vi "临时授权.vi"() -> (3 "授权成功":bool)   [LabVIEW 2019]
panel:
  out "不合格信息":string
  in  "授权":bool
  in  "密码":string
  in  "用户名":string(combo)
  # "产品检测不合格！\n程序已锁定！请联系管理员解除锁定！"
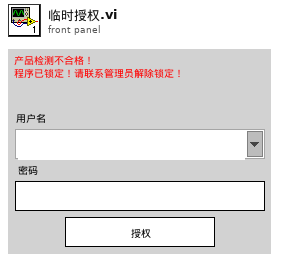
[diagram p1: front panel]
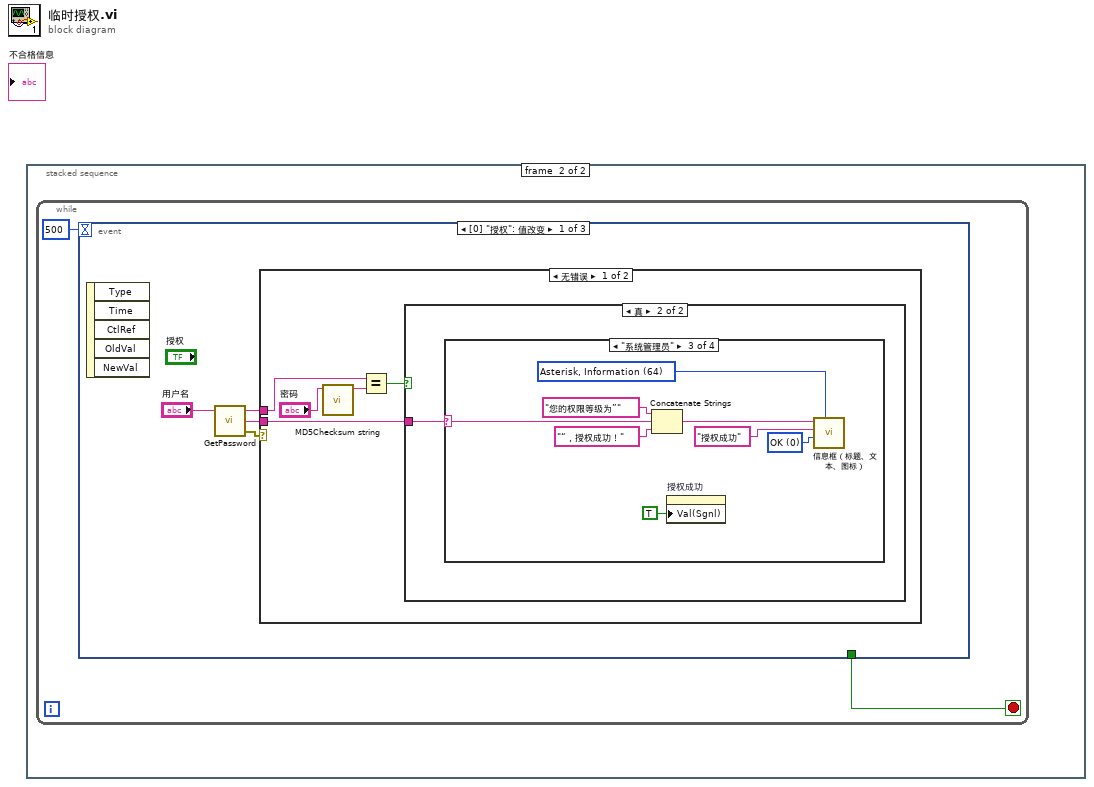
[diagram p0: block diagram]
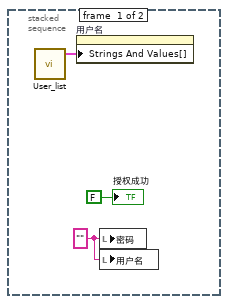
[diagram p2: hidden frame]
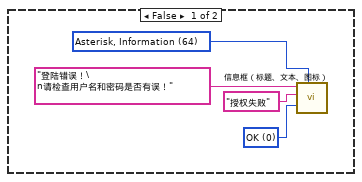
[diagram p3: hidden frame]
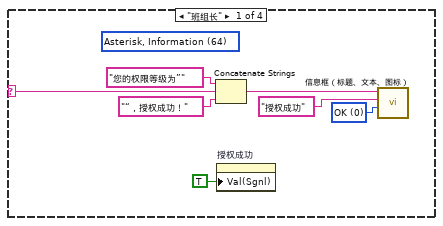
[diagram p4: hidden frame]
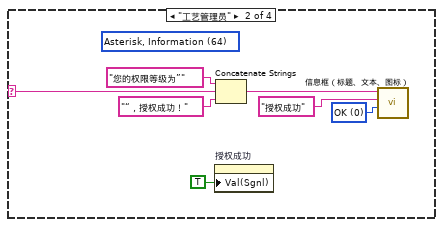
[diagram p5: hidden frame]
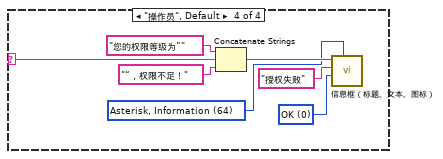
[diagram p6: hidden frame]
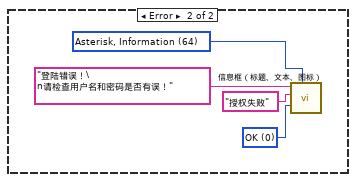
[diagram p7: hidden frame]
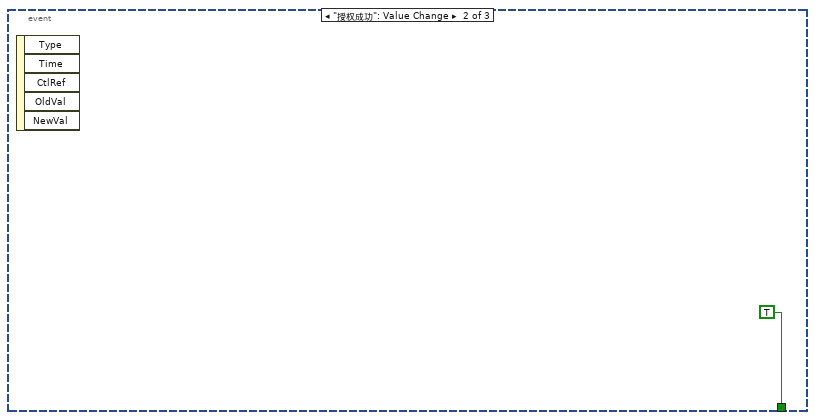
[diagram p8: hidden frame]
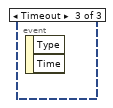
[diagram p9: hidden frame]
diagram:
  n1 = stacked-sequence {
    frame #0 {
      w1 = ""
      n2 = call "User_list.vi"() -> ("User_list"=w3:cluster{string, string}[])  [unwired: 4 in, 1 out]
      n3 = property on="用户名" class="CmbBox"("Strings And Values[]"=w3) -> ()  [unwired: 2 in, 2 out]
      n4 = local write "密码"(w1) -> ()
      n5 = local write "用户名"(w1) -> ()
      "授权成功" <- FALSE ("授权成功")
    }
    frame #1 {
      n6 = while {
        stop <- w4 stop-if-true
        n7 = event shown="[0] \"授权\": 值改变" {
          selector: _ -> [_ _ _]
          dyn-events: _ -> [_ _ _]
          timeout: 500 -> [_ _ _]
          tunnel: [_ TRUE _] -> w4
          event "授权": Value Change {
            n8 = event-data() -> ()  [unwired: 1 in, 5 out]
            n9 = call "GetPassword.vi"("User_Name"="用户名") -> ("error out"=w8:errorcluster, "Permission"=w6:string, "Password"=w7:string)  [unwired: 2 in]
            n10 = case shown="无错误" w8 {
              tunnel: w7 -> [w13 _]
              tunnel: w6 -> [w10 _]
              frame No Error {
                n11 = call <vilib>:"MD5Checksum string.vi"("Message String"="密码") -> ("MD5 message-digest"=w12:string)  [unwired: 10 in]
                n12 = Equal?(x=w13, y=w12) -> (x = y?=w11:bool)
                n13 = case shown="真" w11 {
                  tunnel: w10 -> [_ w19]
                  frame False {
                    w15 = 64 items=["None"=0, "Hand, Error, Stop"=16, "Question"=32, "Exclamation, Warning"=48, "Asterisk, Information"=64] ("icon")
                    w16 = 0 items=["OK", "OKCancel", "AbortRetryIgnore", "YesNoCancel", "YesNo", "RetryCancel"] ("buttons")
                    n14 = call "信息框（标题、文本、图标）.vi"("icon"=w15, "buttons"=w16, "caption"="授权失败", "text"="登陆错误！\n请检查用户名和密码是否有误！") -> ()  [unwired: 6 in, 2 out]
                  }
                  frame True {
                    n15 = case shown="\"系统管理员\"" w19 {
                      selector: w19 -> [w21 w28 w36 w46]
                      frame "班组长" {
                        (unwired) 64 items=["None"=0, "Hand, Error, Stop"=16, "Question"=32, "Exclamation, Warning"=48, "Asterisk, Information"=64] ("icon")
                        w22 = 0 items=["OK", "OKCancel", "AbortRetryIgnore", "YesNoCancel", "YesNo", "RetryCancel"] ("buttons")
                        n16 = Concatenate Strings("您的权限等级为”" ("字符串"), w21, "“，授权成功！" ("字符串")) -> (w23:string)
                        n17 = property on="授权成功" class="Bool (严格)"("Val(Sgnl)"=TRUE ("值(信号)")) -> ()  [unwired: 2 in, 2 out]
                        n18 = call "信息框（标题、文本、图标）.vi"("buttons"=w22, "caption"="授权成功", "text"=w23) -> ()  [unwired: 7 in, 2 out]
                      }
                      frame "工艺管理员" {
                        (unwired) 64 items=["None"=0, "Hand, Error, Stop"=16, "Question"=32, "Exclamation, Warning"=48, "Asterisk, Information"=64] ("icon")
                        w29 = 0 items=["OK", "OKCancel", "AbortRetryIgnore", "YesNoCancel", "YesNo", "RetryCancel"] ("buttons")
                        n19 = property on="授权成功" class="Bool (严格)"("Val(Sgnl)"=TRUE ("值(信号)")) -> ()  [unwired: 2 in, 2 out]
                        n20 = Concatenate Strings("您的权限等级为”" ("字符串"), w28, "“，授权成功！" ("字符串")) -> (w30:string)
                        n21 = call "信息框（标题、文本、图标）.vi"("buttons"=w29, "caption"="授权成功", "text"=w30) -> ()  [unwired: 7 in, 2 out]
                      }
                      frame "系统管理员" {
                        w35 = 64 items=["None"=0, "Hand, Error, Stop"=16, "Question"=32, "Exclamation, Warning"=48, "Asterisk, Information"=64] ("icon")
                        w37 = 0 items=["OK", "OKCancel", "AbortRetryIgnore", "YesNoCancel", "YesNo", "RetryCancel"] ("buttons")
                        n22 = Concatenate Strings("您的权限等级为”" ("字符串"), w36, "“，授权成功！" ("字符串")) -> (w38:string)
                        n23 = property on="授权成功" class="Bool (严格)"("Val(Sgnl)"=TRUE ("值(信号)")) -> ()  [unwired: 2 in, 2 out]
                        n24 = call "信息框（标题、文本、图标）.vi"("icon"=w35, "buttons"=w37, "caption"="授权成功", "text"=w38) -> ()  [unwired: 6 in, 2 out]
                      }
                      frame "操作员", Default {
                        w42 = 64 items=["None"=0, "Hand, Error, Stop"=16, "Question"=32, "Exclamation, Warning"=48, "Asterisk, Information"=64] ("icon")
                        w43 = 0 items=["OK", "OKCancel", "AbortRetryIgnore", "YesNoCancel", "YesNo", "RetryCancel"] ("buttons")
                        n25 = Concatenate Strings("您的权限等级为”" ("字符串"), w46, "“，权限不足！" ("字符串")) -> (w44:string)
                        n26 = call "信息框（标题、文本、图标）.vi"("icon"=w42, "buttons"=w43, "caption"="授权失败", "text"=w44) -> ()  [unwired: 6 in, 2 out]
                      }
                    }
                  }
                }
              }
              frame Error {
                w49 = 64 items=["None"=0, "Hand, Error, Stop"=16, "Question"=32, "Exclamation, Warning"=48, "Asterisk, Information"=64] ("icon")
                w50 = 0 items=["OK", "OKCancel", "AbortRetryIgnore", "YesNoCancel", "YesNo", "RetryCancel"] ("buttons")
                n27 = call "信息框（标题、文本、图标）.vi"("icon"=w49, "buttons"=w50, "caption"="授权失败", "text"="登陆错误！\n请检查用户名和密码是否有误！") -> ()  [unwired: 6 in, 2 out]
              }
            }
          }
          event "授权成功": Value Change {
            n28 = event-data() -> ()  [unwired: 1 in, 5 out]
          }
          event Timeout {
            n29 = event-data() -> ()  [unwired: 1 in, 2 out]
          }
        }
      }
    }
  }
